vi "forceOutputState.vi"(8 "error in (no error)":errorcluster, 9 "data":T1(array[cluster]), 10 "physicalChannels":string[](array[string]), 11 "SpinCore in":refnum<class "SpinCore.lvclass">) -> (0 "error out":errorcluster, 3 "SpinCore out":refnum<class "SpinCore.lvclass">)   [LabVIEW 2011, in "Hardware.lvlib" / "Channels.lvlib" / "SpinCore.lvclass"]
uses:
  SpinCore.lvclass
  SpinCore.lvclass/SpinCore.ctl
  Generic/DDSOutput.lvclass
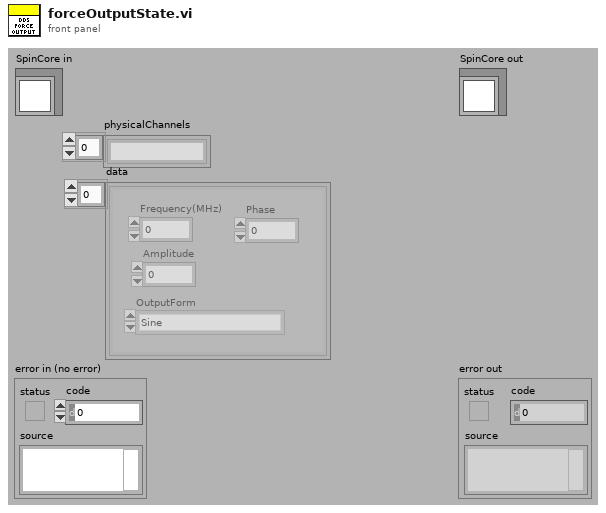
[diagram p1: front panel]
types:
  T1 = cluster{"Frequency(MHz)":dbl, "Amplitude":dbl, "Phase":dbl, "OutputForm":enum16{"Sine", "Square", "Triangle", "Arbitrary"}}[]
  T2 = cluster{"Frequency(MHz)":dbl, "Amplitude":dbl, "Phase":dbl, "OutputForm":enum16{"Sine", "Square", "Triangle", "Arbitrary"}}
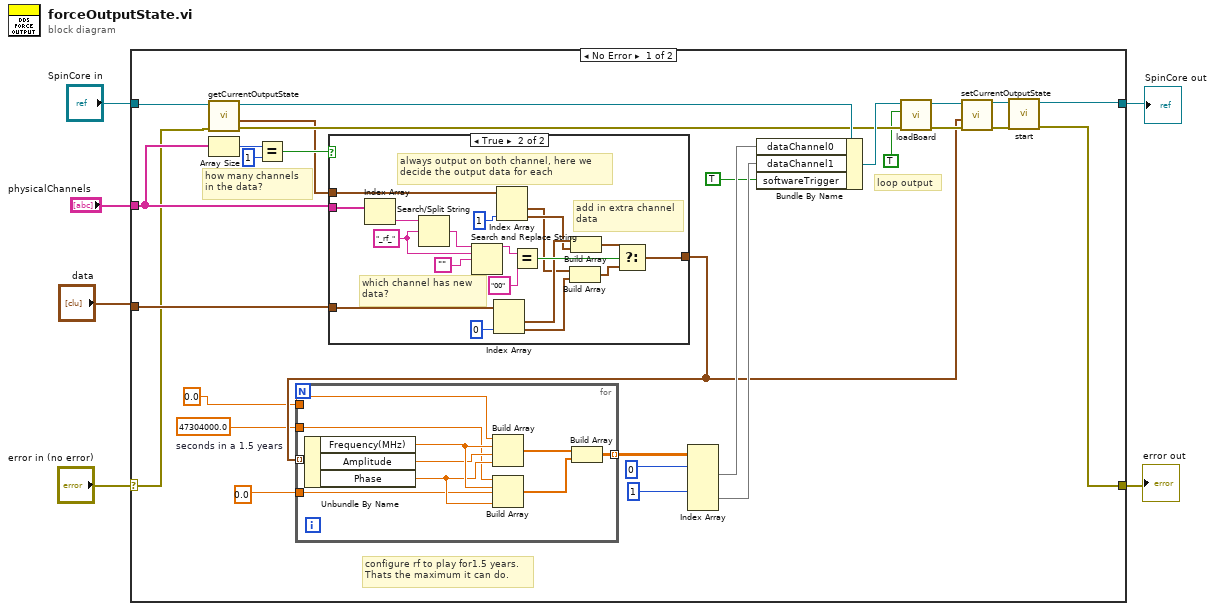
[diagram p0: block diagram]
diagram:
  n1 = case shown="No Error" "error in (no error)" {
    selector: "error in (no error)" -> [w11 w66]
    tunnel: [w27 w65] -> w6
    tunnel: "SpinCore in" -> [w10 w65]
    tunnel: [w26 w66] -> w3
    tunnel: "data" -> [w19 _]
    tunnel: "physicalChannels" -> [w12 _]
    frame No Error {
      w8 = 47304000.0  # seconds in a 1.5 years
      # "configure rf to play for1.5 years.\nThats the maximum it can do."
      # "loop output"
      # "how many channels\nin the data?"
      n2 = call "getCurrentOutputState.vi"("error in (no error)"=w11, "DDSOutput in"=w10) -> ("error out"=w24:errorcluster, "CurrentOutputState"=w20:T1, "DDSOutput out"=w25:refnum<class "SpinCore.lvclass">)  [unwired: 6 in, 1 out]
      n3 = Array Size(array=w12) -> (size(s)=w23:i32)
      n4 = Equal?(x=w23, y=1) -> (x = y?=w21:bool)
      n5 = case shown="True" w21 {
        tunnel: w12 -> [_ w54]
        tunnel: w20 -> [_ w45]
        tunnel: w19 -> [w35 w46]
        tunnel: [w35 w36] -> w14
        frame False {
          # "channels for output will be 2, so no need to enter\ndata for another channel"
        }
        frame True {
          w51 = "_rf_"
          # "add in extra channel\ndata"
          # "which channel has new\ndata?"
          # "always output on both channel, here we\ndecide the output data for each"
          n6 = Index Array(array=w54) -> (element=w53:string)  [unwired: 1 in]
          n7 = Search/Split String(string=w53, search string/char (-)=w51) -> (match + rest of string=w52:string)  [unwired: 1 in, 2 out]
          n8 = Search and Replace String(input string=w52, search string=w51, replace string="") -> (result string=w49:string)  [unwired: 5 in, 3 out]
          n9 = Index Array(array=w46, index #2=0) -> (element #1=w42:T2, element #2=w38:T2)  [unwired: 1 in]
          n10 = Index Array(array=w45, index #2=1) -> (element #1=w39:T2, element #2=w41:T2)  [unwired: 1 in]
          n11 = Equal?(x=w49, y="00") -> (x = y?=w47:bool)
          n12 = Build Array(w39, w38) -> (w37:T1)
          n13 = Build Array(w42, w41) -> (w40:T1)
          n14 = Select(t=w40, s=w47, f=w37) -> (s? t:f=w36:T1)
        }
      }
      n15 = for {
        tunnel: w14 -> [w59] mode=indexing
        tunnel: [w58] -> w34 mode=indexing
        tunnel: 0.0 -> [w57]
        tunnel: w8 -> [w56]
        tunnel: 0.0 -> [w55]
        n16 = Unbundle By Name(w59) -> ("Frequency(MHz)"=w63:dbl, "Amplitude"=w62:dbl, "Phase"=w61:dbl)
        n17 = Build Array(w57, w63, w62, w61) -> (w64:dbl[])
        n18 = Build Array(w56, w63, w55, w61) -> (w60:dbl[])
        n19 = Build Array(w64, w60) -> (w58:dbl[][])
      }
      n20 = Index Array(array=w34, index (dim 0) #1=0, index (dim 0) #2=1) -> (element #1=w31:dbl[][], element #2=w30:dbl[][])  [unwired: 4 in]
      n21 = Bundle By Name(cluster=w25, "dataChannel0"=w31, "dataChannel1"=w30, "softwareTrigger"=TRUE) -> (w29:refnum<class "SpinCore.lvclass">)
      n22 = call "loadBoard.vi"("error in (no error)"=w24, "continuous"=TRUE, "SpinCore in"=w29) -> ("error out"=w17:errorcluster, "SpinCore out"=w18:refnum<class "SpinCore.lvclass">)  [unwired: 7 in]
      n23 = call "setCurrentOutputState.vi"("error in (no error)"=w17, "CurrentOutputState"=w14, "DDSOutput in"=w18) -> ("error out"=w16:errorcluster, "DDSOutput out"=w15:refnum<class "SpinCore.lvclass">)  [unwired: 7 in]
      n24 = call-dynamic "start.vi"("error in (no error)"=w16, "SpinCore in"=w15) -> ("error out"=w26:errorcluster, "SpinCore out"=w27:refnum<class "SpinCore.lvclass">)  [unwired: 8 in]
    }
    frame Error {
    }
  }
  "error out" <- w3
  "SpinCore out" <- w6
